vi "MtAtElectrometer_acceptCommand_setMode.vi"(8 "error in (no error)":errorcluster, 11 "command_setMode_Ctl":T1) -> (0 "error out":errorcluster, 2 "function return":i32, 3 "command_setMode_Ctl out":T1)   [LabVIEW 2016, in "SALLV_MtAtElectrometer.lvlib"]
doc: "int MtAtElectrometer_shm_acceptCommand_setModeLV(MtAtElectrometer_command_setModeLV *command_setMode_Ctl );"
uses:
  SALLV_MtAtElectrometer.lvlib
  DataTypes/command_setMode.ctl
  ts_sal/test/MtAtElectrometer/labview/SALLV_MtAtElectrometer.so
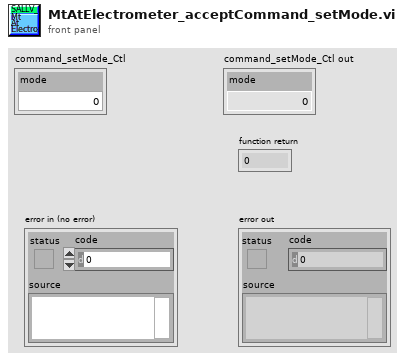
[diagram p1: front panel]
types:
  T1 = typedef "SALLV_MtAtElectrometer.lvlib/command_setMode.ctl" = cluster{"mode":u16}
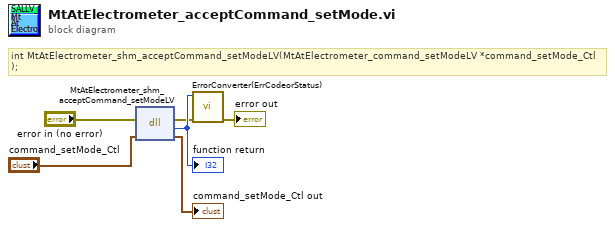
[diagram p0: block diagram]
diagram:
  # "int MtAtElectrometer_shm_acceptCommand_setModeLV(MtAtElectrometer_command_setModeLV *command_setMode_Ctl );"
  n1 = dll-call lib="home/andres/ts_sal/test/MtAtElectrometer/labview/SALLV_MtAtElectrometer.*" fn="MtAtElectrometer_shm_acceptCommand_setModeLV"(error in="error in (no error)", "command_setMode_Ctl"="command_setMode_Ctl") -> (error out=w2:errorcluster, w6:i32, "command_setMode_Ctl"=→"command_setMode_Ctl out":T1)  [unwired: 2 in, 1 out]
  "function return" <- w6
  n2 = call "ErrorConverter(ErrCodeorStatus).vi"("error in (no error)"=w2, "error code"=w6) -> ("error out"=→"error out":errorcluster)  [unwired: 9 in]
